vi "Execute Write Query.vi"(8 "error in (no error)":errorcluster, 10 "Executable In":refnum<class "Executable.lvclass">, 11 "Driver in":refnum<class "Driver.lvclass">) -> (0 "error out":errorcluster, 2 "Executable Out":refnum<class "Executable.lvclass">, 3 "Driver out":refnum<class "Driver.lvclass">)   [LabVIEW 2023, in "HAF.lvlib" / "Driver.lvclass"]
doc: "Using the passed Comman, sends a command to the Instrument.\n\nThere are two methods for this:\n1. Immediate: the command is sent straight to the Instrument.  This is only possible for Commands that Can Overlap\n2. When Able: the Instrument is checked for already running commands and if any, the Command is delayed until the running commands finish."
uses:
  Driver.lvclass
  Driver.lvclass/Driver.ctl
  Executable/Executable.lvclass
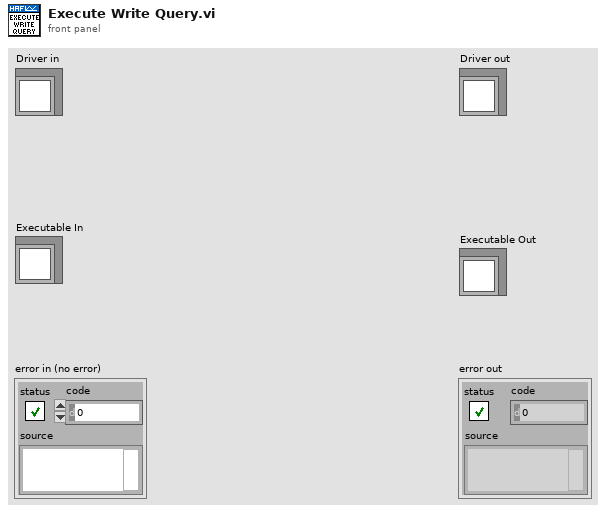
[diagram p1: front panel]
types:
  T1 = cluster{"Can Overlap":bool, "Block on Wait":bool, "Timeout":u32}
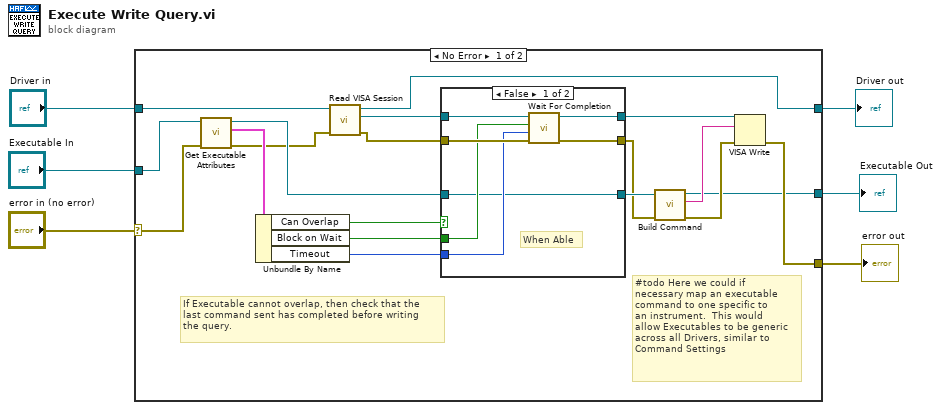
[diagram p0: block diagram]
diagram:
  n1 = case shown="No Error" "error in (no error)" {
    selector: "error in (no error)" -> [w17 w38]
    tunnel: [w10 w38] -> w5
    tunnel: [w8 w37] -> w3
    tunnel: "Driver in" -> [w25 w37]
    tunnel: "Executable In" -> [w23 w36]
    tunnel: [w9 w36] -> w1
    frame No Error {
      # "If Executable cannot overlap, then check that the \nlast command sent has completed before writing\nthe query."
      # "#todo Here we could if\nnecessary map an executable\ncommand to one specific to\nan instrument.  This would\nallow Executables to be generic\nacross all Drivers, similar to\nCommand Settings"
      n2 = call-dynamic "Get Executable Attributes.vi"("error in (no error)"=w17, "Executable in"=w23) -> ("error out"=w16:errorcluster, "Executable Attributes"=w22:T1, "Executable out"=w18:refnum<class "Executable.lvclass">)  [unwired: 7 in]
      n3 = Unbundle By Name(w22) -> ("Can Overlap"=w21:bool, "Block on Wait"=w20:bool, "Timeout"=w19:u32)
      n4 = call-dynamic "Read VISA Session.vi"("error in (no error)"=w16, "Driver in"=w25) -> ("error out"=w7:errorcluster, "VISA Session"=w24:refnum<visa-resource-name>, "Driver out"=w8:refnum<class "Driver.lvclass">)  [unwired: 7 in]
      n5 = case shown="False" w21 {
        tunnel: w18 -> [w26 w33]
        tunnel: w24 -> [w32 w35]
        tunnel: w7 -> [w31 w34]
        tunnel: [w30 w35] -> w13
        tunnel: [w29 w34] -> w14
        tunnel: [w26 w33] -> w15
        tunnel: w20 -> [w28 _]
        tunnel: w19 -> [w27 _]
        frame False {
          # "When Able"
          n6 = call "Wait For Completion.vi"("error in (no error)"=w31, "Timeout"=w27, "Block on Wait"=w28, "Session In"=w32) -> ("error out"=w29:errorcluster, "Session Out"=w30:refnum<visa-resource-name>)  [unwired: 6 in]
        }
        frame True {
          # "Immediate - no need to wait"
        }
      }
      n7 = call-dynamic "Build Command.vi"("error in (no error)"=w14, "Executable in"=w15) -> ("error out"=w11:errorcluster, "Command"=w12:string, "Executable out"=w9:refnum<class "Executable.lvclass">)  [unwired: 7 in]
      n8 = VISA Write(VISA resource name=w13, write buffer=w12, error in (no error)=w11) -> (error out=w10:errorcluster)  [unwired: 2 out]
    }
    frame Error {
    }
  }
  "error out" <- w5
  "Driver out" <- w3
  "Executable Out" <- w1
